vi "libdaq_gpio_read_port.vi"(0 "error in (no error)":errorcluster, 1 "device_name":string, 2 "module_name":string) -> (14 "error out":errorcluster, 15 "device_name":string, 16 "module_name":string, 18 "portval":bool[](array[boolean]))   [LabVIEW 2010, in "libdaqVI.lvlib"]
doc: "读取一个GPIO模块所有IO的状态，当该GPIO模块的某些IO配置为“OUT”或者“AF”模式时，将自动忽略对该IO的读取操作，因此返回的相应IO数据是无效的"
uses:
  libdaqVI.lvlib
  dll/daqlib.dll
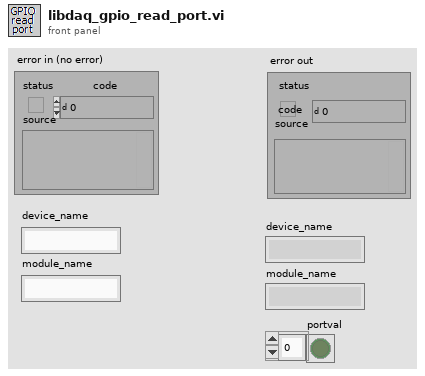
[diagram p1: front panel]
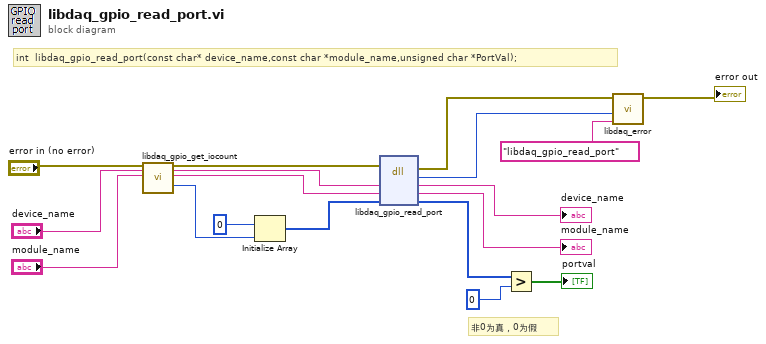
[diagram p0: block diagram]
diagram:
  # "非0为真，0为假"
  # "int  libdaq_gpio_read_port(const char* device_name,const char *module_name,unsigned char *PortVal);"
  n1 = call "libdaq_gpio_get_iocount.vi"("error in (no error)"="error in (no error)", "device_name"="device_name", "module_name"="module_name") -> ("error out"=w15:errorcluster, "device_name"=w12:string, "module_name"=w11:string, "iocount"=w10:u8)  [unwired: 13 in]
  n2 = Initialize Array(u8 0, w10) -> (w17:u8[])
  n3 = dll-call lib="E:/Product/Example/DAQ-USB3212/Labview/labview_2010/libdaqVI/dll/daqlib.dll" fn="libdaq_gpio_read_port"(error in=w15, "device_name"=w12, "module_name"=w11, "PortVal"=w17) -> (error out=w9:errorcluster, "return type"=w7:i32, "device_name"=→"device_name":string, "module_name"=→"module_name":string, "PortVal"=w5:u8[])  [unwired: 2 in, 1 out]
  n4 = Greater?(x=w5, y=u8 0) -> (0:→"portval":bool[])
  n5 = call "libdaq_error.vi"("error source"="libdaq_gpio_read_port", "error code"=w7, "错误输入（无错误）"=w9) -> ("错误输出"=→"error out":errorcluster)  [unwired: 8 in]
